vi "AWG Select and Initiate Multiple Scripts.vi"(6 "Timeout (msec)":i32=50000, 8 "error in (no error)":errorcluster, 10 "script names":string[](array[string]), 11 "Semiconductor Module Context":T1) -> (0 "error out":errorcluster, 2 "Sessions Out":refnum<k15>[](array[refnum]), 3 "Semiconductor Module Context Out":T1)   [LabVIEW 2013]
doc: "Selects and initiates the script name selected."
uses:
  <vilib>/NI_TestStand_SemiconductorModule/NI_TestStand_Semiconductor_Module.lvlibp/PinMap/General/SemiconductorModuleContext.ctl
  <vilib>/NI_TestStand_SemiconductorModule/NI_TestStand_Semiconductor_Module.lvlibp
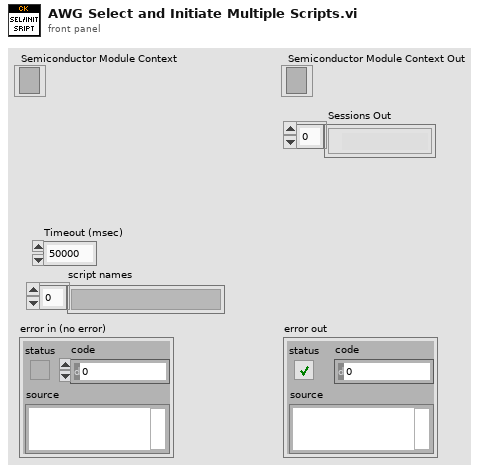
[diagram p1: front panel]
types:
  T1 = typedef "NI_TestStand_Semiconductor_Module.lvlibp/SemiconductorModuleContext.ctl" = refnum<k7>
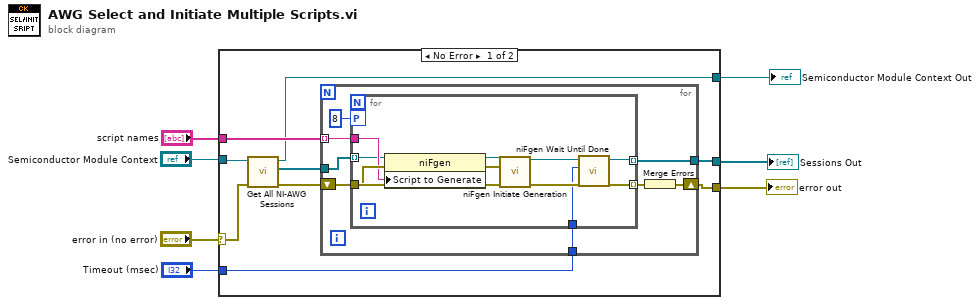
[diagram p0: block diagram]
diagram:
  n1 = case shown="No Error" "error in (no error)" {
    selector: "error in (no error)" -> [w12 w35]
    tunnel: "Semiconductor Module Context" -> [w10 w34]
    tunnel: "script names" -> [w16 _]
    tunnel: [w15 w35] -> w1
    tunnel: [w14 _] -> w2
    tunnel: "Timeout (msec)" -> [w9 _]
    tunnel: [w8 w34] -> w4
    frame No Error {
      n2 = call "Get All NI-AWG Sessions.vi"("error in (no error)"=w12, "Semiconductor Module Context"=w10) -> ("error out"=w13:errorcluster, "Instrument Sessions"=w11:refnum<k15>[], "Semiconductor Module Context Out"=w8:T1)  [unwired: 7 in]
      n3 = for {
        tunnel: w16 -> [w23] mode=indexing
        tunnel: [w21] -> w14
        tunnel: w11 -> [w19]
        tunnel: w9 -> [w18]
        shift-right: [w22] -> w15
        shift-left: w13 -> [w17]
        n4 = for {
          tunnel: w17 -> [w33]
          tunnel: w23 -> [w30]
          tunnel: [w27] -> _ mode=indexing
          tunnel: [w28] -> w21 mode=indexing
          workers-P: 8 -> [_]
          tunnel: w19 -> [w29] mode=indexing
          tunnel: w18 -> [w24]
          n5 = property class="niFgen"(reference=w29, error in=w33, "Script to Generate"=w30) -> (reference out=w31:refnum<k15>, error out=w32:errorcluster)
          n6 = call <instrlib>:"niFgen Initiate Generation.vi"("error in (no error)"=w32, "Instrument Handle"=w31) -> ("error out"=w25:errorcluster, "Instrument Handle Out"=w26:refnum<k15>)  [unwired: 8 in]
          n7 = call <instrlib>:"niFgen Wait Until Done.vi"("error in (no error)"=w25, "MaxTime (msec)"=w24, "Instrument Handle"=w26) -> ("error out"=w27:errorcluster, "Instrument Handle Out"=w28:refnum<k15>)  [unwired: 7 in]
        }
        n8 = Merge Errors(w17) -> (w22:errorcluster)
      }
    }
    frame Error {
    }
  }
  "error out" <- w1
  "Sessions Out" <- w2
  "Semiconductor Module Context Out" <- w4
